vi "Set Wavelength.vi"(8 "error in (no error)":errorcluster, 10 "Wavelength (nm)":dbl, 11 "SpectraPro in":refnum<class "SpectraPro.lvclass">) -> (0 "error out":errorcluster, 2 "Wavelength (nm) out":dbl, 3 "SpectraPro out":refnum<class "SpectraPro.lvclass">)   [LabVIEW 2019, in "SpectraPro.lvclass"]
uses:
  SpectraPro.lvclass
  SpectraPro.lvclass/SpectraPro.ctl
  SpectraPro-LabVIEW-Driver/SpectraPro.lvlib
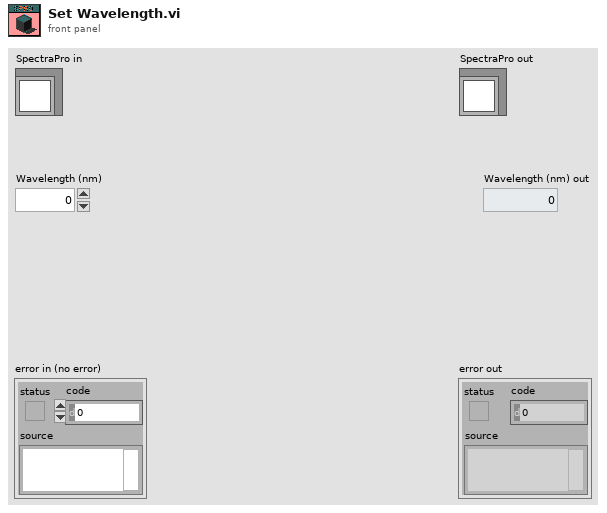
[diagram p1: front panel]
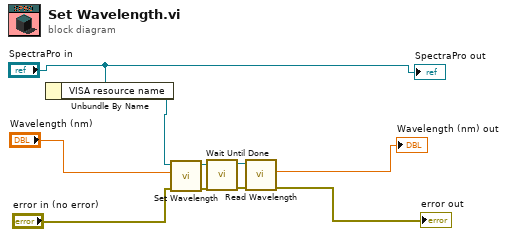
[diagram p0: block diagram]
diagram:
  n1 = Unbundle By Name("SpectraPro in") -> ("VISA resource name"=w9:refnum<visa-resource-name>)
  n2 = call "Set Wavelength.vi"("error in (no error)"="error in (no error)", "Wavelength (nm)"="Wavelength (nm)", "VISA resource name"=w9) -> ("error out"=w7:errorcluster, "VISA resource name out"=w6:refnum<visa-resource-name>)  [unwired: 6 in, 1 out]
  n3 = call "Wait Until Done.vi"("error in (no error)"=w7, "VISA resource name"=w6) -> ("error out"=w5:errorcluster, "VISA resource name out"=w4:refnum<visa-resource-name>)  [unwired: 8 in]
  n4 = call "Read Wavelength.vi"("error in (no error)"=w5, "VISA resource name"=w4) -> ("error out"=→"error out":errorcluster, "Wavelength (nm)"=→"Wavelength (nm) out":dbl)  [unwired: 6 in, 2 out]
  "SpectraPro out" <- "SpectraPro in"
